vi "Get Classes Names.vi"() -> (3 "class name":string[](array[string]))   [LabVIEW 2020, in "Osciloscope Tektronix.lvlib"]
uses:
  Osciloscope Tektronix.lvlib
  Clases/Osciloscope/Osciloscope.lvclass
  Clases/Tektonix 2000/Tektonix 2000.lvclass
  Clases/EDUX1002G/EDUX1002G.lvclass
  C:/Users/Pablo/Osciloscope-Tek/TDS2000/Libraries/Osciloscope Tektronix/Clases/Osciloscope/Osciloscope.lvclass
panel:
  in  "Ring":u16(ring)
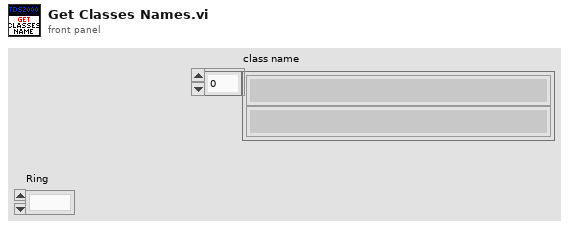
[diagram p1: front panel]
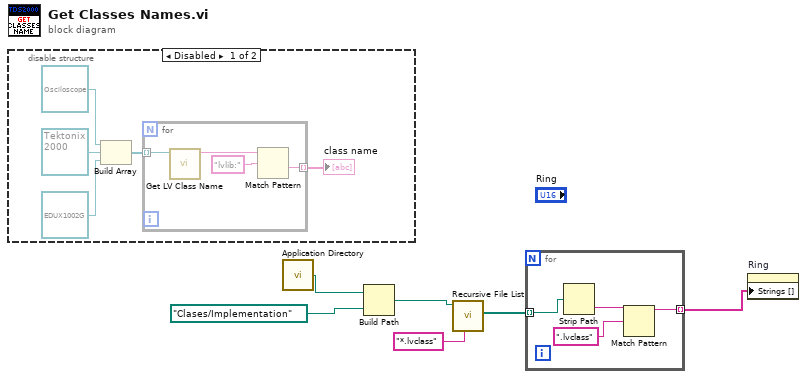
[diagram p0: block diagram]
diagram:
  n1 = disable-structure shown="Disabled" {
    frame Disabled {
      n2 = Build Array(refnum<class "Osciloscope.lvclass"> refnum ("Osciloscope Tektronix.lvlib:Osciloscope.lvclass"), refnum<class "Tektonix 2000.lvclass"> refnum ("Osciloscope Tektronix.lvlib:Tektonix 2000.lvclass"), refnum<class "EDUX1002G.lvclass"> refnum ("Osciloscope Tektronix.lvlib:EDUX1002G.lvclass")) -> (w10:refnum<class "Osciloscope.lvclass">[])
      n3 = for {
        tunnel: w10 -> [w15] mode=indexing
        tunnel: [w13] -> w8 mode=indexing
        n4 = call <vilib>:"Get LV Class Name.vi"("object"=w15) -> ("class name"=w14:string)  [unwired: 9 in, 1 out]
        n5 = Match Pattern(string=w14, regular expression="lvlib:") -> (after substring=w13:string)  [unwired: 1 in, 3 out]
      }
      "class name" <- w8
    }
    frame Enabled {
    }
  }
  n6 = call <vilib>:"Application Directory.vi"() -> ("Application Directory"=w5:path)
  n7 = Build Path(base path=w5, name or relative path=path "Clases/Implementation") -> (appended path=w4:path)
  n8 = call <vilib>:"Recursive File List.vi"("pattern"="*.lvclass", "Folder Path"=w4) -> ("All Files in Dir"=w2:path[])  [unwired: 5 in, 4 out]
  n9 = for {
    tunnel: w2 -> [w18] mode=indexing
    tunnel: [w16] -> w1 mode=indexing
    n10 = Strip Path(path=w18) -> (name=w19:string)  [unwired: 1 out]
    n11 = Match Pattern(string=w19, regular expression=".lvclass") -> (before substring=w16:string)  [unwired: 1 in, 3 out]
  }
  n12 = property on="Ring" class="Ring (strict)"("Strings []"=w1) -> ()  [unwired: 2 in, 2 out]
